vi "Update Sinks Event Handlers Dict.vi"(0 "Event Source in":refnum<class "Event Source.lvclass">, 1 "Sink Enququer":refnum<class "Message Enqueuer.lvclass">, 2 "Exclude From Broadcast (F)":bool, 3 "Paused (F)":bool, 5 "error in (no error)":errorcluster) -> (14 "Event Source out":refnum<class "Event Source.lvclass">, 19 "error out":errorcluster)   [LabVIEW 2016, in "Event Source.lvlib" / "Event Source.lvclass"]
uses:
  Event Source.lvclass
  <vilib>/ActorFramework/Message Enqueuer/Message Enqueuer.lvclass
  Event Source.lvclass/Event Source.ctl
  Event Handler Details.ctl
  Event Source Messages/Event Generated Msg/Event Generated Msg.lvclass
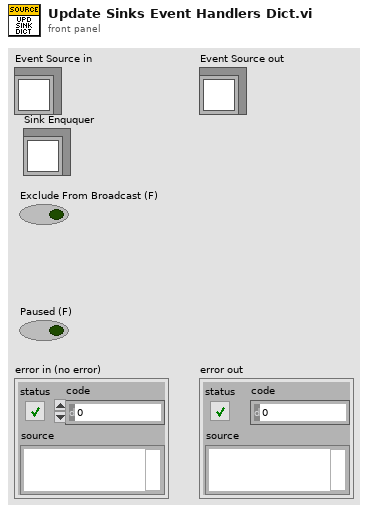
[diagram p1: front panel]
types:
  T1 = typedef "Event Source.lvlib/Event Source.lvclass/Event Handler Details.ctl" = cluster{"Exclude From Broadcast":bool, "Paused":bool, "Sink Event Fire Handler":refnum<class "Event Generated Msg.lvclass">}
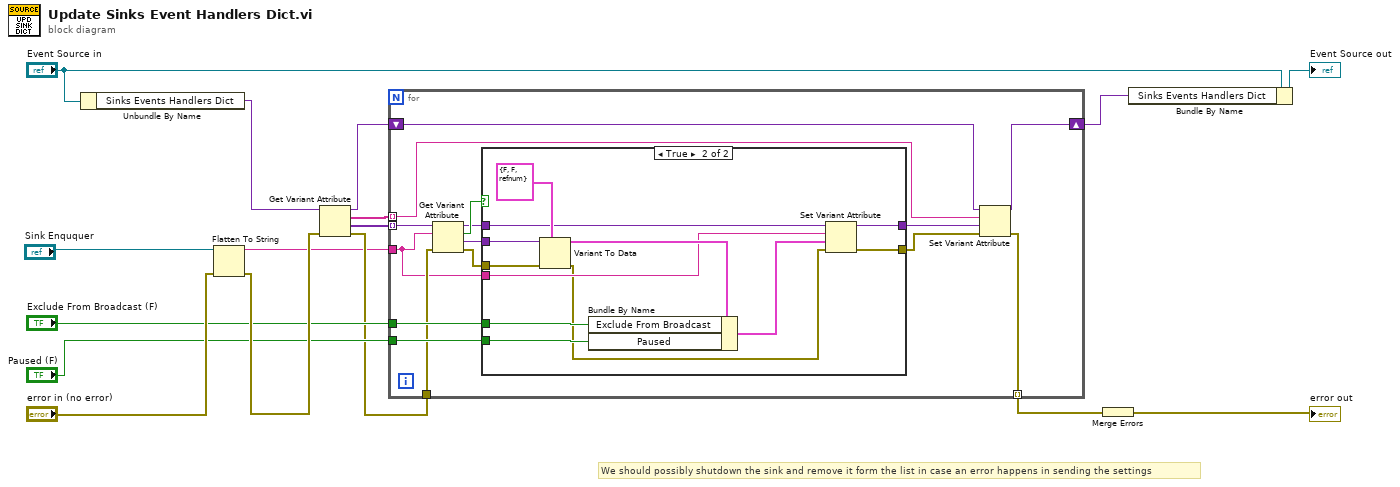
[diagram p0: block diagram]
diagram:
  # "We should possibly shutdown the sink and remove it form the list in case an error happens in sending the settings"
  n1 = Unbundle By Name("Event Source in") -> ("Sinks Events Handlers Dict"=w14:variant)
  n2 = Flatten To String(anything="Sink Enququer", error in (no error)="error in (no error)") -> (data string=w6:string, error out=w11:errorcluster)  [unwired: 2 in, 1 out]
  n3 = Get Variant Attribute(Variant=w14, error in=w11) -> (duplicate Variant=w2:variant, names=w4:string[], values=w8:variant[], error out=w7:errorcluster)  [unwired: 2 in]
  n4 = for {
    tunnel: "Exclude From Broadcast (F)" -> [w31]
    tunnel: "Paused (F)" -> [w30]
    tunnel: w8 -> [w29] mode=indexing
    tunnel: w7 -> [w28]
    tunnel: w6 -> [w24]
    tunnel: [w20] -> w5 mode=indexing
    tunnel: w4 -> [w22] mode=indexing
    shift-right: [w18] -> w3
    shift-left: w2 -> [w17]
    n5 = Get Variant Attribute(Variant=w29, name=w24, error in=w28) -> (duplicate Variant=w23:variant, found=w27:bool, value=w26:variant, error out=w25:errorcluster)  [unwired: 1 in]
    n6 = case shown="True" w27 {
      tunnel: w31 -> [_ w45]
      tunnel: w30 -> [_ w44]
      tunnel: w26 -> [_ w43]
      tunnel: w25 -> [w32 w41]
      tunnel: w24 -> [_ w39]
      tunnel: w23 -> [w33 w37]
      tunnel: [w32 w35] -> w19
      tunnel: [w33 w34] -> w21
      frame False {
      }
      frame True {
        n7 = Variant To Data(error in=w41, type=T1 {"Exclude From Broadcast"=FALSE, "Paused"=FALSE, "Sink Event Fire Handler"=refnum} ("Event Handler Details"), Variant=w43) -> (data=w40:T1, error out=w38:errorcluster)
        n8 = Bundle By Name(cluster=w40, "Exclude From Broadcast"=w45, "Paused"=w44) -> (w36:T1)
        n9 = Set Variant Attribute(Variant=w37, name=w39, value=w36, error in=w38) -> (Variant out=w34:variant, error out=w35:errorcluster)  [unwired: 1 out]
      }
    }
    n10 = Set Variant Attribute(Variant=w17, name=w22, value=w21, error in=w19) -> (Variant out=w18:variant, error out=w20:errorcluster)  [unwired: 1 out]
  }
  n11 = Merge Errors(w5) -> (→"error out":errorcluster)
  n12 = Bundle By Name(cluster="Event Source in", "Sinks Events Handlers Dict"=w3) -> (→"Event Source out":refnum<class "Event Source.lvclass">)
